vi "Termo_1.5__.vi"() -> ()   [LabVIEW 2013]
doc: "Программа мониторинга температуры"
uses:
  <vilib>/Utility/error.llb/DialogType.ctl
  Global R.vi
  Global T.vi
  Global P.vi
  PV ActiveLine/PV ActiveLine.lvlib
panel:
  out "Sensor 2":dbl format="%.3e"
  out "Sensor 1":dbl format="%.3e"
  in  "TPG COM port":refnum<visa-resource-name> caption="Eingang (Referenz)"
  in  "Интервал сохр. в файл, мин":u32=2 caption="Интервал сохр. в файл"
  out "Err":string=" INSTRUCTIONS:\r\rNormal Use:  When using subVIs that incorporate the error in/error out (or error I/O) structure, place this handler where you want to inform the user of an error, typically at the end of the I/O data path, as the last action of the program.  If the error in error? is ERROR, the handler creates a message describing the error and its source.  If the type of dialog = 1 (default), the message is displayed to the user, who can only acknowedge it.  If the type = 2, the user can acknowledge the message or abort execution; aborting a program with active I/O is not recommended.  If the type = 0, no message is displayed; this is used to process the error programmatically, and the error out cluster elements are wired to individual terminals for that reason.  \r\rOther Use:\n\r\nlocal testing.  To test the error code of a subVI or function that does not have the error I/O structure, you can wire its error code and a source string to the local error code and error source inputs.  If error in error? indicates no error and error code is not equal to 0, the local code and source are substituted for the error in values, and error? is set TRUE (ERROR)."
  out "Status Sensor 2":i32(ring) items=["data OK", "underrange", "overrange", "sensor error", "sensor off", "no sensor", "ID error"]
  out "Status Sensor 1":i32(ring) items=["data OK", "underrange", "overrange", "sensor error", "sensor off", "no sensor", "ID error"]
  in  "T13 koeff.":T1={"k1"=26.4009671199601144, "k2"=-324.931044271681458, "k3"=1711.37684206105769, "k4"=-4392.68239063024521, "k5"=6058.41654951870441, "k6"=-3986.95889506489038, "k7"=1183.01099493727087997} {"k7" format="%#_18g"; "k6" format="%#_18g"; "k5" format="%#_18g"; "k4" format="%#_18g"; "k3" format="%#_18g"; "k2" format="%#_18g"; "k1" format="%#_18g"}
  in  "T12 koeff.":T1={"k1"=17.07349405885907, "k2"=-214.441047532483935, "k3"=1210.98502247408031995, "k4"=-3244.2372938580811, "k5"=4710.0469546467065798, "k6"=-3214.85599070042372, "k7"=997.561462182551622} {"k7" format="%#_18g"; "k6" format="%#_18g"; "k5" format="%#_18g"; "k4" format="%#_18g"; "k3" format="%#_18g"; "k2" format="%#_18g"; "k1" format="%#_18g"}
  in  "T11 koeff.":T1={"k1"=23.375991559296380701, "k2"=-279.282885558437556, "k3"=1443.09818702377379, "k4"=-3601.37313615530729, "k5"=4833.89744386076927, "k6"=-3091.9414890073239801, "k7"=931.25663803331553903} {"k7" format="%#_18g"; "k6" format="%#_18g"; "k5" format="%#_18g"; "k4" format="%#_18g"; "k3" format="%#_18g"; "k2" format="%#_18g"; "k1" format="%#_18g"}
  in  "T10 koeff.":T1={"k1"=14.2047637495270465, "k2"=-178.266357081010938, "k3"=1036.21158173121512, "k4"=-2804.05543357878923, "k5"=4109.27601800113916, "k6"=-2758.27630065754056, "k7"=841.102514177560806} {"k7" format="%#_18g"; "k6" format="%#_18g"; "k5" format="%#_18g"; "k4" format="%#_18g"; "k3" format="%#_18g"; "k2" format="%#_18g"; "k1" format="%#_18g"}
  in  "T8 koeff.":T1={"k1"=22.4768360081361607, "k2"=-287.193510523065925, "k3"=1596.74034120887518, "k4"=-4282.5984272807836502, "k5"=6172.9084560498595202, "k6"=-4207.9212595894932698, "k7"=1298.64862929470837005} {"k7" format="%#_18g"; "k6" format="%#_18g"; "k5" format="%#_18g"; "k4" format="%#_18g"; "k3" format="%#_18g"; "k2" format="%#_18g"; "k1" format="%#_18g"}
  in  "T7 koeff.":T1={"k1"=22.696802702761488001, "k2"=-226.07392810517922, "k3"=970.613756582140923, "k4"=-1955.80814630538225, "k5"=2022.28153763338923, "k6"=-904.462546051479876, "k7"=215.64549227920360901} {"k7" format="%#_18g"; "k6" format="%#_18g"; "k5" format="%#_18g"; "k4" format="%#_18g"; "k3" format="%#_18g"; "k2" format="%#_18g"; "k1" format="%#_18g"}
  in  "T6 koeff.":T1={"k1"=28.2578839106718078, "k2"=-358.860014421865344, "k3"=1945.6722907833755, "k4"=-5171.24013045430183, "k5"=7400.41584329307079, "k6"=-5088.91018018126488, "k7"=1538.68586002103984} {"k7" format="%#_18g"; "k6" format="%#_18g"; "k5" format="%#_18g"; "k4" format="%#_18g"; "k3" format="%#_18g"; "k2" format="%#_18g"; "k1" format="%#_18g"}
  in  "T5 koeff.":T1={"k1"=11.9987486686586634996, "k2"=-140.311366179957986, "k3"=706.404515956528485, "k4"=-1587.81046432070434005, "k5"=1758.85326032713056, "k6"=-724.664392888546, "k7"=148.42783740232699} {"k7" format="%#_18g"; "k6" format="%#_18g"; "k5" format="%#_18g"; "k4" format="%#_18g"; "k3" format="%#_18g"; "k2" format="%#_18g"; "k1" format="%#_18g"}
  in  "T4 koeff.":T1={"k1"=35.418606627499684698, "k2"=-55510.2443863153458, "k3"=36541155.640991210901, "k4"=-11725993248.921875, "k5"=1971553990780.0, "k6"=-153283011720960.0, "k7"=5052534013419520.0} {"k7" format="%#_18g"; "k6" format="%#_18g"; "k5" format="%#_18g"; "k4" format="%#_18g"; "k3" format="%#_18g"; "k2" format="%#_18g"; "k1" format="%#_18g"}
  in  "T3 koeff.":T1={"k1"=25.230552436260040799, "k2"=-268.022426915355027, "k3"=1234.06186301074921996, "k4"=-2752.2769357189536099, "k5"=3276.3375887721777, "k6"=-1820.06986418552697, "k7"=447.66889524366706599} {"k7" format="%#_18g"; "k6" format="%#_18g"; "k5" format="%#_18g"; "k4" format="%#_18g"; "k3" format="%#_18g"; "k2" format="%#_18g"; "k1" format="%#_18g"}
  in  "T2 koeff.":T1={"k1"=21.575617982307449, "k2"=-260.23302811570465001, "k3"=1369.9472036678344, "k4"=-3472.20134520530701, "k5"=4749.71195641905069, "k6"=-3111.58472899347544, "k7"=957.900049353018403} {"k7" format="%#_18g"; "k6" format="%#_18g"; "k5" format="%#_18g"; "k4" format="%#_18g"; "k3" format="%#_18g"; "k2" format="%#_18g"; "k1" format="%#_18g"}
  in  "T1 koeff.":T1={"k1"=16.924520218221005099, "k2"=-209.88193494221195599, "k3"=1166.48439995385706, "k4"=-3075.28152279928327, "k5"=4388.5694366171956098, "k6"=-2910.95083422213793, "k7"=868.100233905948699} {"k7" format="%#_18g"; "k6" format="%#_18g"; "k5" format="%#_18g"; "k4" format="%#_18g"; "k3" format="%#_18g"; "k2" format="%#_18g"; "k1" format="%#_18g"}
  out "R16":dbl format="%.2f"
  out "R15":dbl format="%.2f"
  out "PKT2 updated":bool=TRUE
  out "PKT1 updated":bool=TRUE
  out "ПКТ2-R":T2
  out "ПКТ2-T":T2
  out "ПКТ1-T":T2
  out "ПКТ1-R":T2
  in  "Графики N температур":bool
  in  "4 K gr":bool
  in  "Tab Control":enum32{"Измерения", "Настройки"}(tab)
  in  "stop":bool
  out "R9":dbl format="%.2f"
  out "R10":dbl format="%.2f"
  out "R11":dbl format="%.2f"
  out "R12":dbl format="%.2f"
  out "R13":dbl format="%.2f"
  out "R14":dbl format="%.2f"
  out "R7":dbl format="%.2f"
  out "R5":dbl format="%.2f"
  out "R8":dbl format="%.2f"
  out "R6":dbl format="%.2f"
  out "R3":dbl format="%.2f"
  out "R1":dbl format="%.2f"
  out "R4":dbl format="%.2f"
  out "R2":dbl format="%.2f"
  in  "GraphLookB":bool
  in  "Старт измер.":bool
  in  "Стоп измер.":bool
  in  "IP-адрес 2":string="192.168.127.102"
  in  "порт 2":u16=4001
  in  "connect 2":bool
  in  "disconnect 2":bool
  in  "порт":u16=4001
  in  "IP-адрес":string="192.168.127.101"
  in  "connect":bool
  in  "disconnect":bool
  in  "SPS":T3(ring)
  in  "Buf_size":u8=16 min=1 max=128
  in  "ADC_dyn_range":T4(ring)=enum."± 0.625 В"
  out "Связь с прибором":bool
  out "Связь с прибором 2":bool
  out "Т7":dbl format="%.2f"
  out "Т1":dbl format="%.2f"
  out "T12":dbl format="%.2f"
  out "T10":dbl format="%.2f"
  out "T9":dbl format="%.2f"
  out "T11":dbl format="%.2f"
  out "T13":dbl format="%.2f"
  out "T14":dbl format="%.2f"
  out "Т8":dbl format="%.2f"
  out "Т6":dbl format="%.2f"
  out "Т5":dbl format="%.2f"
  out "T4":dbl format="%.2f"
  out "Т2":dbl format="%.2f"
  out "Т3":dbl format="%.2f"
  out "T15":dbl format="%.2f"
  out "T16":dbl format="%.2f"
  out "connection ID 2":refnum<k5>
  out "disconnected 2":bool
  out "Расположение\n файла":path caption="Расположение файла"
  in  "load_coeff.":bool caption="Disconn"
  in  "save_coeff.":bool caption="Disconn"
  out "Configuring ADC?":bool
  in  "Запись в файл":bool
  out "refnum out":refnum<file>
  in  "File header exist?":bool caption="Disconn"
  out "connection ID":refnum<k5>
  out "Расположение файла":path
  # "КРИОН-Т"
  # "4 K"
  # "40 K"
  # "P"
  # "mBar"
  # "мин."
  # "Измерения"
  # "R [Ом]"
  # "R1"
  # "R2"
  # "R3"
  # "R4"
  # "R5"
  # "R6"
  # "R7"
  # "R8"
  # "R9"
  # "R10"
  # "R11"
  # "R12"
  # "R13"
  # "R14"
  # "Скорость измерений"
  # "SPS = Samples Per Second"
  # "Динамический диапазон"
  # "Размер буфера усреднения"
  # "Подключение"
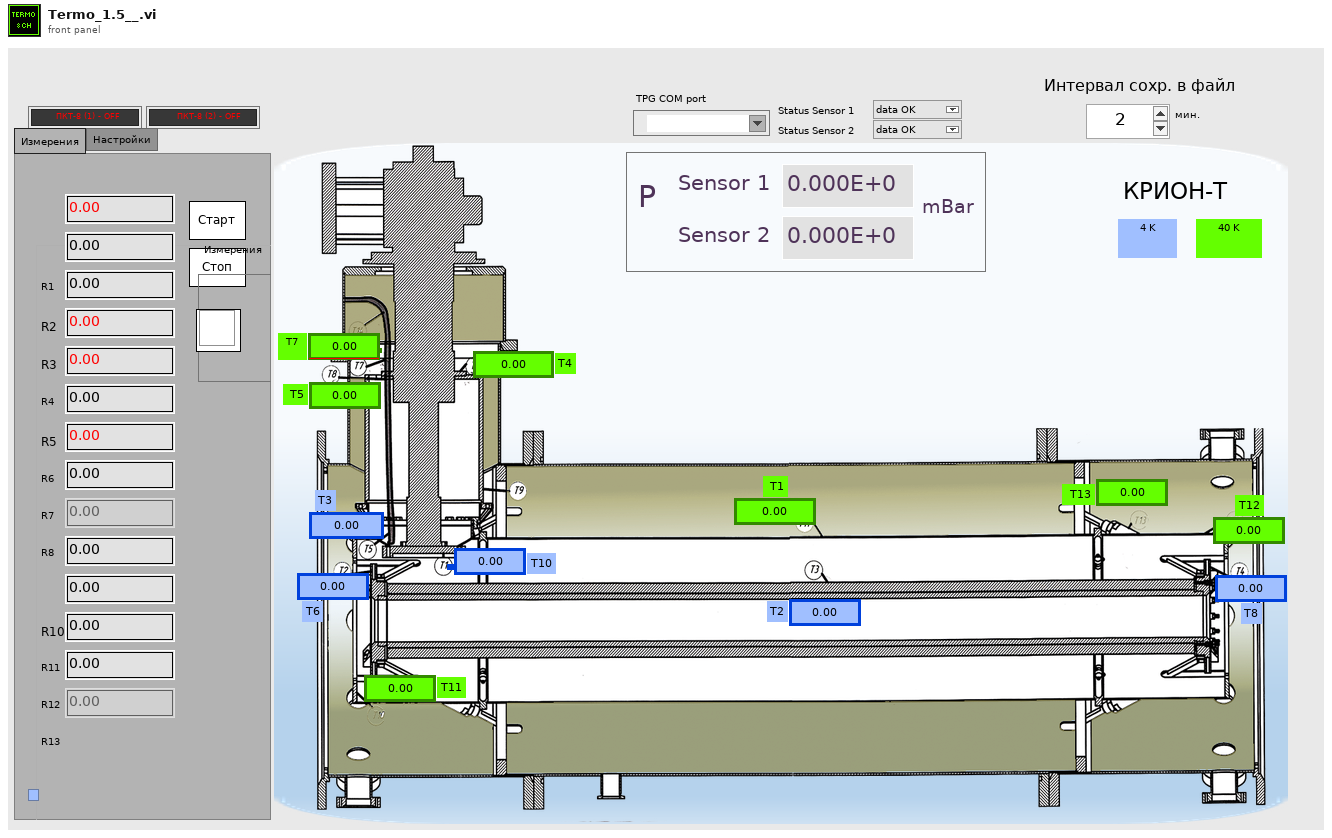
[diagram p1: front panel]
types:
  T1 = cluster{"k1":ext, "k2":ext, "k3":ext, "k4":ext, "k5":ext, "k6":ext, "k7":ext}
  T2 = cluster{" R1":dbl, " R2":dbl, " R3":dbl, " R4":dbl, " R5":dbl, "R6":dbl, " R7":dbl, "R8":dbl}
  T3 = enum16{"2,5 SPS", "5 SPS", "10 SPS", "25 SPS", "50 SPS", "100 SPS", "500 SPS", "1 kSPS", "3,75 kSPS"}
  T4 = enum16{"± 5 В", "± 2.5 В", "± 1.25 В", "± 0.625 В", "± 312.5 мВ", "± 156.25 мВ", "± 78.125 мВ"}
  T5 = enum32{"Page Enabled", "Page Disabled", "Page Disabled & Grayed"}
  T6 = typedef "DialogType.ctl" = u16
  T7 = enum16{"Standard", "Buffered", "CRLF", "Immediate"}
  T8 = cluster{"Pressure Sensor 1":dbl, "Pressure Sensor 2":dbl}
  T9 = cluster{" R9":dbl, " R10":dbl, " R11":dbl, " R12":dbl, " R13":dbl, "R14":dbl, "R15":dbl, "R16":dbl}
  T10 = cluster{" T9":dbl, "T10":dbl, "T11":dbl, "T12":dbl, " T13":dbl, "T14":dbl, "T15":dbl, "T16":dbl}
  T11 = cluster{" R1":dbl, " R2":dbl, " R3":dbl, " R4":dbl, " R5":dbl, "R6":dbl, " R7":dbl, "R8":dbl, " R1":dbl, " R2":dbl, " R3":dbl, " R4":dbl, " R5":dbl, "R6":dbl, " R7":dbl, "R8":dbl}
  T12 = cluster{" Т1":dbl, "Т2":dbl, "Т3":dbl, "T4":dbl, " Т5":dbl, "Т6":dbl, "Т7":dbl, "Т8":dbl}
  T13 = enum32{"Invalid", "Standard", "Closed", "Hidden", "Minimized", "Maximized"}
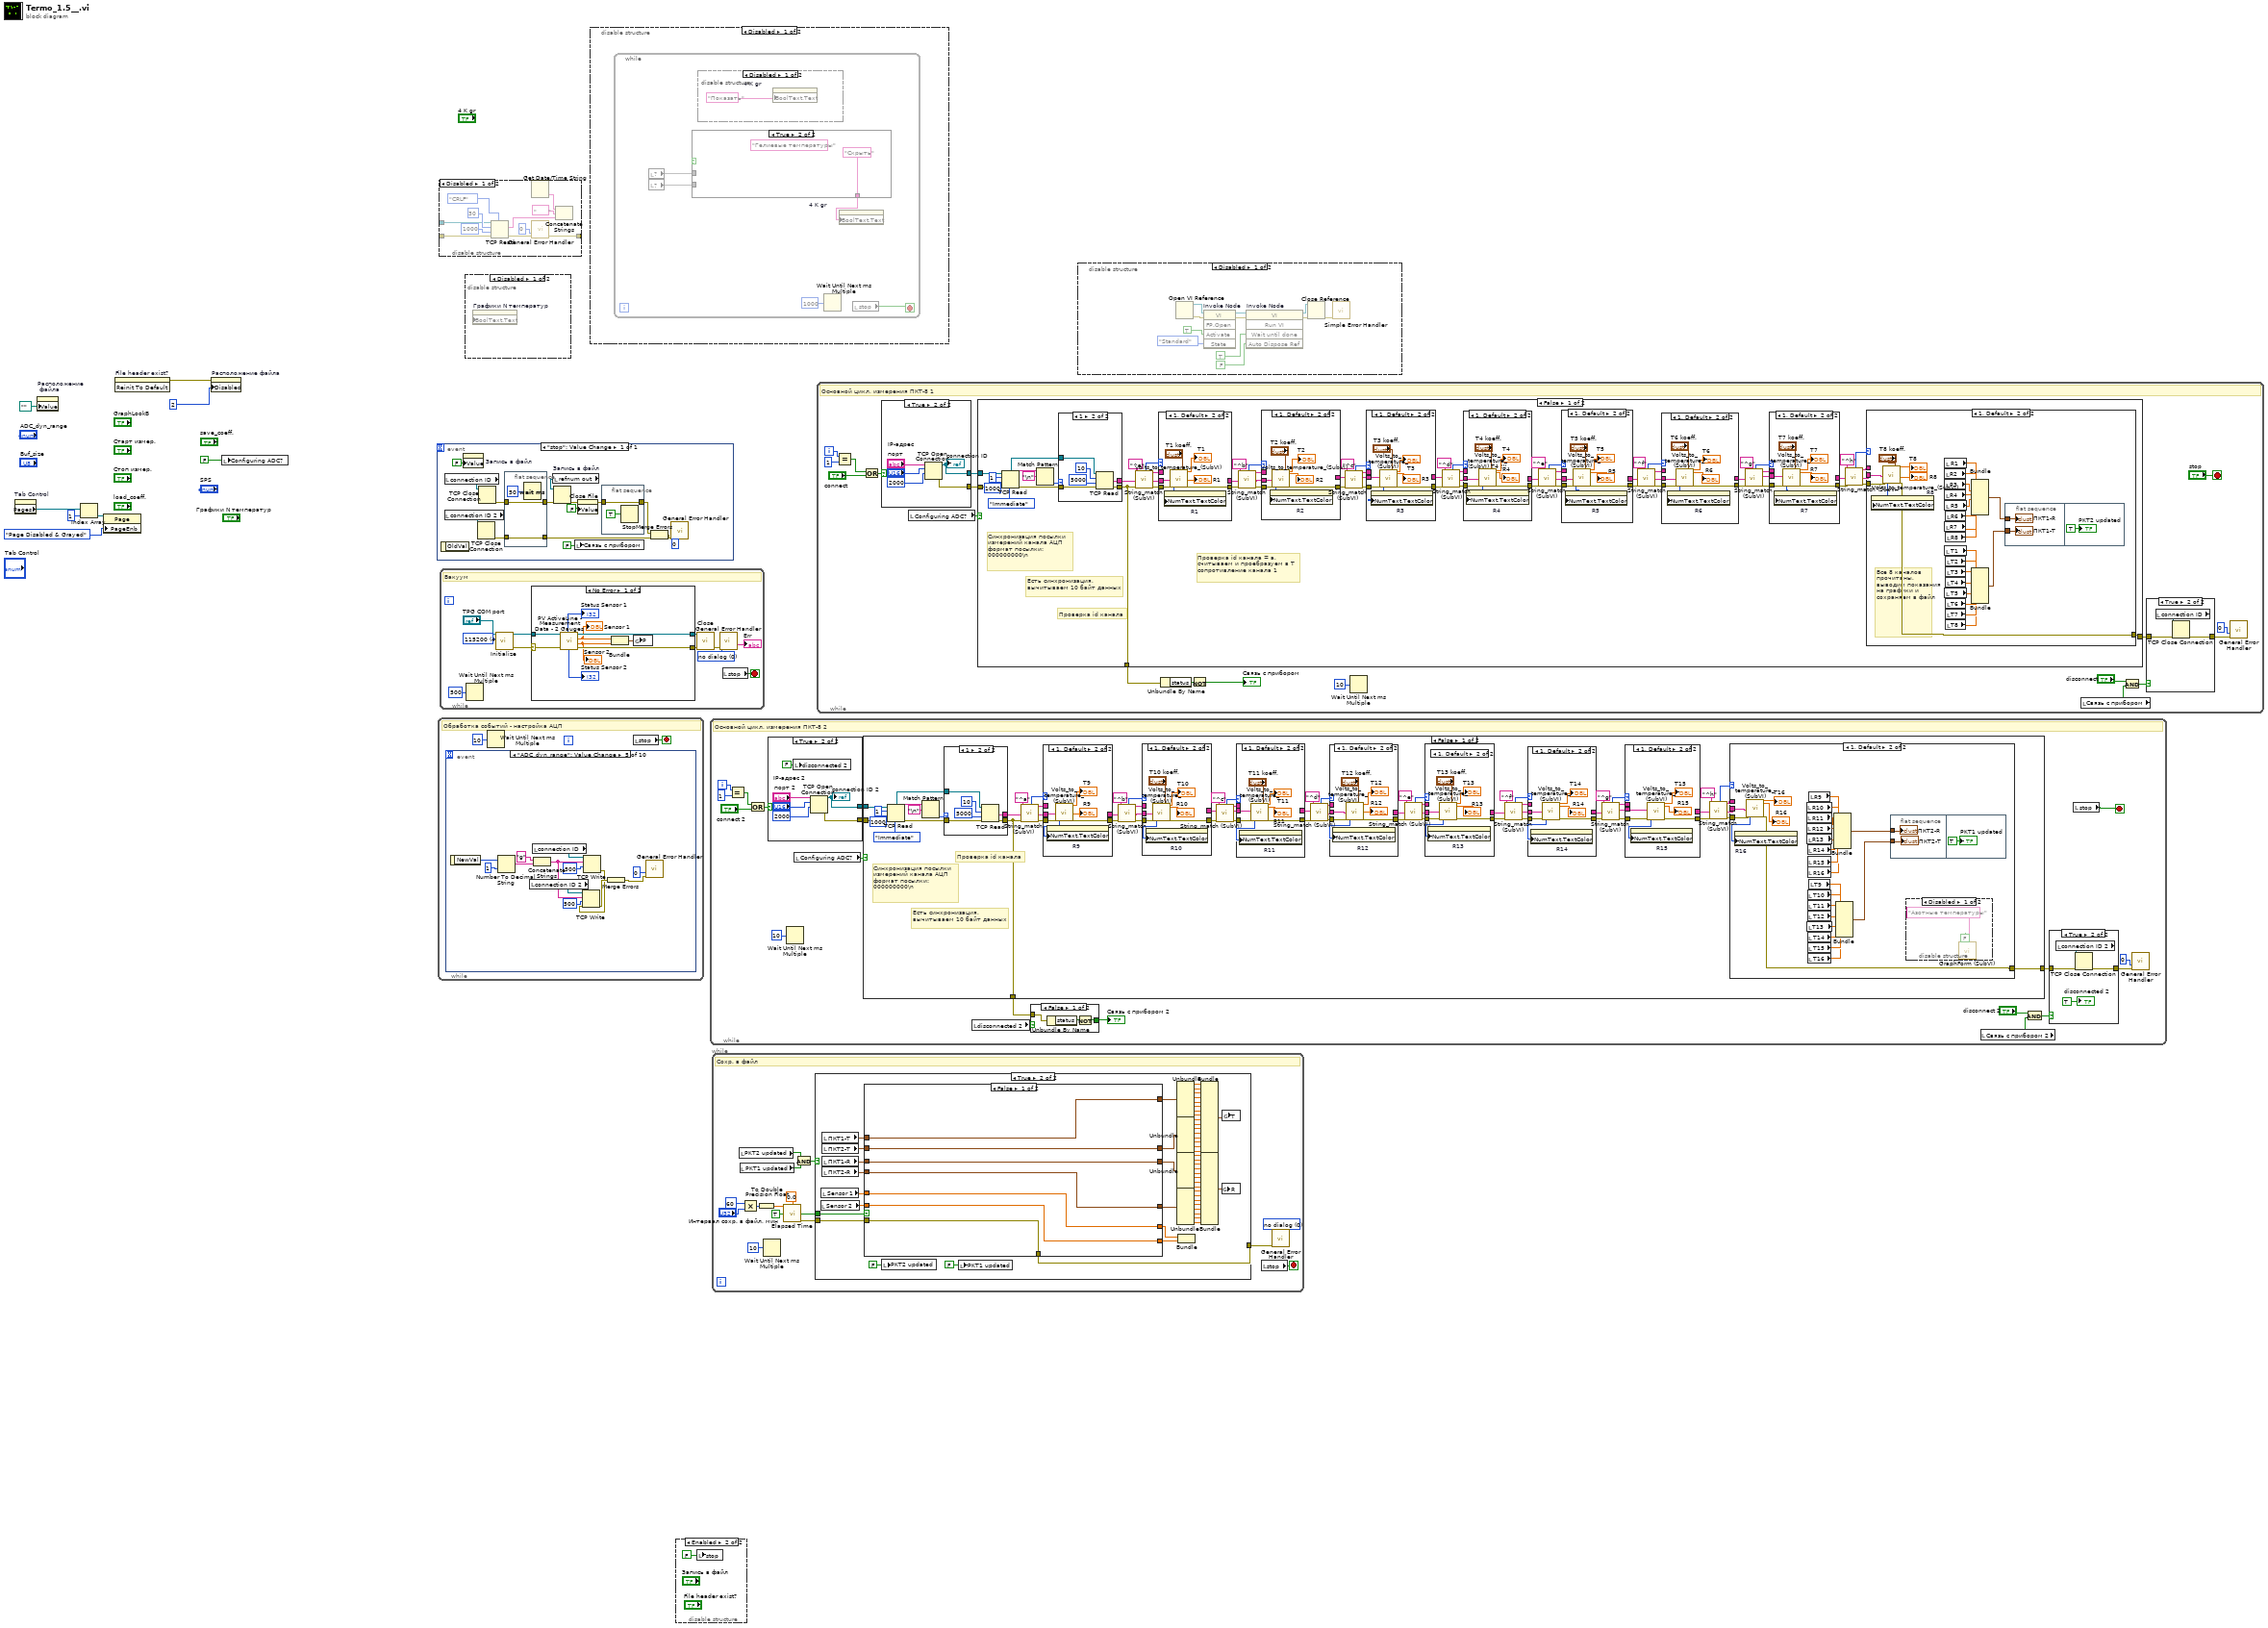
[diagram p0: block diagram]
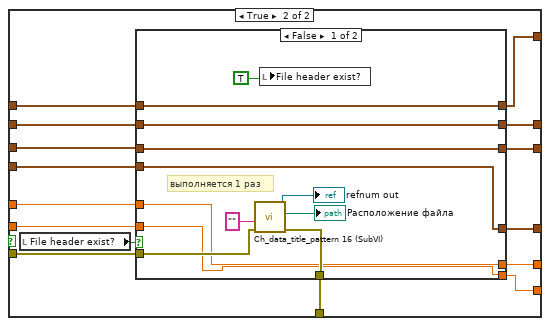
[diagram p3: hidden frame]
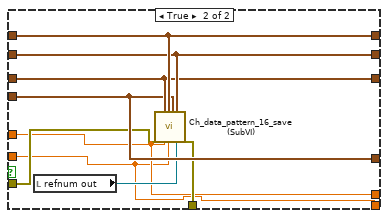
[diagram p4: hidden frame]
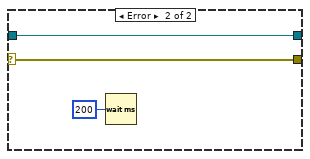
[diagram p5: hidden frame]
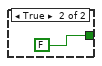
[diagram p8: hidden frame]
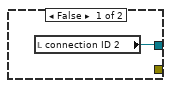
[diagram p10: hidden frame]
diagram:
  n1 = property on="Tab Control" class="TabCtl (strict)"() -> ("Pages"=w1:refnum<vi>[])  [unwired: 2 in, 2 out]
  n2 = property on="Расположение\n файла" class="Path"("Value"=path "" ("Расположение\n файла")) -> ()  [unwired: 2 in, 2 out]
  n3 = Index Array(array=w1, index=1) -> (element=w3:refnum<vi>)
  n4 = property class="Page"(reference=w3, "PageEnb"=T5."Page Disabled & Grayed" ("Page Enabled State")) -> ()  [unwired: 1 in, 2 out]
  n5 = invoke on="File header exist?" class="Bool (strict)" method="Reinit To Default"() -> (error out=w7:errorcluster)  [unwired: 3 in, 2 out]
  n6 = property on="Расположение файла" class="Path"(error in=w7, "Disabled"=u8 2) -> ()  [unwired: 1 in, 2 out]
  n7 = local write "Configuring ADC?"(FALSE ("TCP_Wr_fl")) -> ()
  n8 = event shown="[0] \"stop\": Value Change" {
    selector: _ -> [_]
    dyn-events: _ -> [_]
    timeout: _ -> [_]
    event "stop": Value Change {
      (unwired) 0 ("timeout ms (25000)")
      n9 = event-data() -> ()  [unwired: 1 in, 1 out]
      n10 = local read "connection ID"() -> (w17:refnum<k5>)
      n11 = local read "connection ID 2"() -> (w15:refnum<k5>)
      n12 = property on="Запись в файл" class="Bool (strict)"("Value"=FALSE ("Запись в файл")) -> ()  [unwired: 2 in, 2 out]
      n13 = TCP Close Connection(connection ID=w15) -> (error out=w14:errorcluster)  [unwired: 1 in, 2 out]
      n14 = TCP Close Connection(connection ID=w17) -> (error out=w22:errorcluster)  [unwired: 1 in, 2 out]
      n15 = flat-sequence {
        tunnel: [w26] -> w12
        tunnel: w22 -> [w26]
        tunnel: [w25] -> w11
        tunnel: w14 -> [w25]
        frame #0 {
          n16 = Wait (ms)(milliseconds to wait=u32 50) -> ()  [unwired: 1 out]
        }
      }
      n17 = local read "refnum out"() -> (w19:refnum<file>)
      n18 = Close File(refnum=w19, error in=w12) -> (error out=w18:errorcluster)  [unwired: 1 out]
      n19 = local write "Связь с прибором"(FALSE ("Запись в файл")) -> ()
      n20 = property on="Запись в файл" class="Bool (strict)"(error in=w18, "Value"=FALSE ("Запись в файл")) -> (error out=w16:errorcluster)  [unwired: 1 in, 1 out]
      n21 = flat-sequence {
        tunnel: w16 -> [w24]
        tunnel: [w24] -> w10
        frame #0 {
          n22 = Stop(stop? (T)=TRUE) -> ()
        }
      }
      n23 = Merge Errors(w10, w11) -> (w13:errorcluster)
      n24 = call <vilib>:"General Error Handler.vi"("error in (no error)"=w13) -> ()  [unwired: 10 in, 5 out]
    }
  }
  n25 = while {
    stop <- w28 stop-if-true
    # "Обработка событий - настройка АЦП"
    n26 = event shown="[4] \"ADC_dyn_range\": Value Change" {
      selector: _ -> [_ _ _ _ _ _ _ _ _ _]
      dyn-events: _ -> [_ _ _ _ _ _ _ _ _ _]
      timeout: _ -> [_ _ _ _ _ _ _ _ _ _]
      event "Старт измер.": Value Change {
        w37 = 0.0 ("3")
        w41 = 0.0 ("3")
        n27 = event-data() -> ("OldVal"=w49:bool)  [unwired: 1 in]
        n28 = local write "Старт измер."(w49) -> ()
        n29 = local read "connection ID"() -> (w45:refnum<k5>)
        n30 = local read "connection ID 2"() -> (w36:refnum<k5>)
        n31 = property on="Tab Control" class="TabCtl (strict)"() -> (error out=w39:errorcluster, "Pages"=w38:refnum<vi>[])  [unwired: 2 in, 1 out]
        n32 = Index Array(array=w38, index=1) -> (element=w44:refnum<vi>)
        n33 = local write "R3"(w41) -> ()
        n34 = local write "R8"(w41) -> ()
        n35 = local write "R1"(w41) -> ()
        n36 = local write "R6"(w41) -> ()
        n37 = local write "R4"(w41) -> ()
        n38 = local write "R2"(w41) -> ()
        n39 = local write "R5"(w41) -> ()
        n40 = local write "R7"(w41) -> ()
        n41 = property class="Page"(reference=w44, error in=w39, "PageEnb"=T5."Page Disabled & Grayed" ("Page Enabled State")) -> (error out=w32:errorcluster)  [unwired: 1 out]
        n42 = TCP Write(connection ID=w45, data in="s", 9:500 ("timeout ms (25000)")) -> (error out=w30:errorcluster)  [unwired: 1 in, 2 out]
        n43 = TCP Write(connection ID=w36, data in="s", error in (no error)=w30, 9:500 ("timeout ms (25000)")) -> (error out=w33:errorcluster)  [unwired: 2 out]
        n44 = local write "R10"(w37) -> ()
        n45 = local write "R11"(w37) -> ()
        n46 = local write "R12"(w37) -> ()
        n47 = local write "R13"(w37) -> ()
        n48 = local write "R14"(w37) -> ()
        n49 = local write "R15"(w37) -> ()
        n50 = local write "R16"(w37) -> ()
        n51 = local write "R9"(w37) -> ()
        n52 = Merge Errors(w33, w32) -> (w31:errorcluster)
        n53 = call <vilib>:"General Error Handler.vi"("type of dialog (OK msg:1)"=0 ("timeout ms (25000)"), "error in (no error)"=w31) -> ()  [unwired: 9 in, 5 out]
        "Configuring ADC?" <- FALSE ("TCP_Wr_fl")
      }
      event "Стоп измер.": Value Change {
        n54 = event-data() -> ("OldVal"=w67:bool)  [unwired: 1 in]
        n55 = local read "connection ID 2"() -> (w58:refnum<k5>)
        n56 = property on="Tab Control" class="TabCtl (strict)"() -> (error out=w51:errorcluster, "Pages"=w59:refnum<vi>[])  [unwired: 2 in, 1 out]
        n57 = local read "connection ID"() -> (w64:refnum<k5>)
        n58 = local write "Configuring ADC?"(TRUE ("TCP_Wr_fl")) -> ()
        n59 = local write "Стоп измер."(w67) -> ()
        n60 = Index Array(array=w59, index=1) -> (element=w62:refnum<vi>)
        n61 = property class="Page"(reference=w62, error in=w51, "PageEnb"=T5."Page Enabled" ("Page Enabled State")) -> (error out=w52:errorcluster)  [unwired: 1 out]
        n62 = TCP Write(connection ID=w64, data in="p", 9:500 ("timeout ms (25000)")) -> (error out=w50:errorcluster)  [unwired: 1 in, 2 out]
        n63 = TCP Write(connection ID=w58, data in="p", error in (no error)=w50, 9:500 ("timeout ms (25000)")) -> (error out=w53:errorcluster)  [unwired: 2 out]
        n64 = Merge Errors(w53, w52) -> (w54:errorcluster)
        n65 = call <vilib>:"General Error Handler.vi"("type of dialog (OK msg:1)"=0 ("timeout ms (25000)"), "error in (no error)"=w54) -> ()  [unwired: 9 in, 5 out]
      }
      event "SPS": Value Change {
        n66 = event-data() -> ("NewVal"=w76:T3)  [unwired: 1 in]
        n67 = Number To Decimal String(number=w76, width (-)=i16 1) -> (decimal integer string=w74:string)
        n68 = Concatenate Strings("v" ("data in"), w74) -> (w70:string)
        n69 = local read "connection ID 2"() -> (w72:refnum<k5>)
        n70 = local read "connection ID"() -> (w78:refnum<k5>)
        n71 = TCP Write(connection ID=w78, data in=w70, 9:500 ("timeout ms (25000)")) -> (error out=w69:errorcluster)  [unwired: 1 in, 2 out]
        n72 = TCP Write(connection ID=w72, data in=w70, error in (no error)=w69, 9:500 ("timeout ms (25000)")) -> (error out=w68:errorcluster)  [unwired: 2 out]
        n73 = call <vilib>:"General Error Handler.vi"("type of dialog (OK msg:1)"=0 ("timeout ms (25000)"), "error in (no error)"=w68) -> ()  [unwired: 9 in, 5 out]
      }
      event "Buf_size": Value Change {
        n74 = event-data() -> ("NewVal"=w94:u8)  [unwired: 1 in]
        n75 = Number To Decimal String(number=w94, width (-)=i16 3) -> (decimal integer string=w92:string)
        n76 = Concatenate Strings("b" ("data in"), w92) -> (w91:string)
        n77 = call <vilib>:"Space Constant.vi"() -> ("String"=w90:string)
        n78 = Search and Replace String(replace all?=TRUE ("replace all? (F)"), input string=w91, search string=w90, replace string="0" ("replace string (\"\")")) -> (result string=w81:string, error out=w87:errorcluster)  [unwired: 4 in, 2 out]
        n79 = local read "connection ID 2"() -> (w85:refnum<k5>)
        n80 = local read "connection ID"() -> (w96:refnum<k5>)
        n81 = TCP Write(connection ID=w96, data in=w81, error in (no error)=w87, 9:500 ("timeout ms (25000)")) -> (error out=w80:errorcluster)  [unwired: 2 out]
        n82 = TCP Write(connection ID=w85, data in=w81, error in (no error)=w80, 9:500 ("timeout ms (25000)")) -> (error out=w83:errorcluster)  [unwired: 2 out]
        n83 = Merge Errors(w83) -> (w82:errorcluster)
        n84 = call <vilib>:"General Error Handler.vi"("type of dialog (OK msg:1)"=0 ("timeout ms (25000)"), "error in (no error)"=w82) -> ()  [unwired: 9 in, 5 out]
      }
      event "ADC_dyn_range": Value Change {
        n85 = event-data() -> ("NewVal"=w107:T4)  [unwired: 1 in]
        n86 = Number To Decimal String(number=w107, width (-)=i16 1) -> (decimal integer string=w105:string)
        n87 = local read "connection ID 2"() -> (w103:refnum<k5>)
        n88 = local read "connection ID"() -> (w109:refnum<k5>)
        n89 = Concatenate Strings("g" ("data in"), w105) -> (w99:string)
        n90 = TCP Write(connection ID=w109, data in=w99, 9:500 ("timeout ms (25000)")) -> (error out=w98:errorcluster)  [unwired: 1 in, 2 out]
        n91 = TCP Write(connection ID=w103, data in=w99, error in (no error)=w98, 9:500 ("timeout ms (25000)")) -> (error out=w101:errorcluster)  [unwired: 2 out]
        n92 = Merge Errors(w101) -> (w100:errorcluster)
        n93 = call <vilib>:"General Error Handler.vi"("type of dialog (OK msg:1)"=0 ("timeout ms (25000)"), "error in (no error)"=w100) -> ()  [unwired: 9 in, 5 out]
      }
      event "save_coeff.": Value Change {
        w111 = T6 0 items=["no dialog", "OK message", "continue or stop message", "OK message + warnings", "continue/stop + warnings"] ("type of dialog (OK msg:1)")
        n94 = event-data() -> ("OldVal"=w115:bool)  [unwired: 1 in]
        n95 = call "Cluster_to_string_(SubVI).vi"() -> ("string of coefficients"=w119:string, "error out"=w114:errorcluster)  [unwired: 14 in]
        n96 = call "Cluster_to_string_(SubVI).vi"() -> ("string of coefficients"=w120:string, "error out"=w113:errorcluster)  [unwired: 14 in]
        n97 = local write "save_coeff."(w115) -> ()
        n98 = Concatenate Strings(w119, w120) -> (w116:string)
        n99 = Merge Errors(w114, w113) -> (w118:errorcluster)
        n100 = call "Create_and_save_to_file (SubVI).vi"("input string"=w116, "error in"=w118) -> ("Текущее расположение файла"=→"Расположение\n файла":path, "error out"=w112:errorcluster)  [unwired: 4 in]
        n101 = call <vilib>:"General Error Handler.vi"("type of dialog (OK msg:1)"=w111, "error in (no error)"=w112) -> ()  [unwired: 9 in, 5 out]
      }
      event "load_coeff.": Value Change {
        w122 = T6 0 items=["no dialog", "OK message", "continue or stop message", "OK message + warnings", "continue/stop + warnings"] ("type of dialog (OK msg:1)")
        n102 = event-data() -> ("OldVal"=w128:bool)  [unwired: 1 in]
        n103 = Read from Text File(prompt (Open existing file)="Укажите  файл с коэффициентами...") -> (refnum out=w121:refnum<file>, text=w125:string, cancelled=w124:bool, error out=w126:errorcluster)  [unwired: 3 in]
        n104 = case shown="False" w124 {
          tunnel: w126 -> [w140 w141]
          tunnel: w125 -> [w139 _]
          tunnel: [w129 w141] -> w123
          tunnel: w121 -> [w131 _]
          frame False {
            n105 = call "String_to_num (SubVI).vi"("String in"=w139, "error in"=w140) -> ("Rest of string OUT"=w138:string)  [unwired: 5 in, 2 out]
            n106 = Refnum to Path(1:w131) -> (0:w130:path)
            n107 = call "String_to_num (SubVI).vi"("String in"=w138) -> ("Rest of string OUT"=w137:string)  [unwired: 6 in, 2 out]
            n108 = call "String_to_num (SubVI).vi"("String in"=w137) -> ("Rest of string OUT"=w136:string)  [unwired: 6 in, 2 out]
            n109 = local write "Расположение\n файла"(w130) -> ()
            n110 = call "String_to_num (SubVI).vi"("String in"=w136) -> ("Rest of string OUT"=w135:string)  [unwired: 6 in, 2 out]
            n111 = call "String_to_num (SubVI).vi"("String in"=w135) -> ("Rest of string OUT"=w134:string)  [unwired: 6 in, 2 out]
            n112 = call "String_to_num (SubVI).vi"("String in"=w134) -> ("Rest of string OUT"=w133:string)  [unwired: 6 in, 2 out]
            n113 = call "String_to_num (SubVI).vi"("String in"=w133) -> ("Rest of string OUT"=w132:string)  [unwired: 6 in, 2 out]
            n114 = call "String_to_num (SubVI).vi"("String in"=w132) -> ("error out"=w129:errorcluster)  [unwired: 6 in, 2 out]
          }
          frame True {
          }
        }
        n115 = local write "load_coeff."(w128) -> ()
        n116 = call <vilib>:"General Error Handler.vi"("type of dialog (OK msg:1)"=w122, "error in (no error)"=w123) -> ()  [unwired: 9 in, 5 out]
      }
      event "GraphLookB": Value Change {
        n117 = event-data() -> ()  [unwired: 1 in, 1 out]
        n118 = control-ref of="This VI"() -> (w142:refnum<vi>)
        n119 = local write "GraphLookB"(FALSE ("Снимок")) -> ()
        n120 = call "CheckScreenShot (SubVI).vi"("VI reference"=w142) -> ()  [unwired: 15 in]
      }
      event "4 K gr": Value Change {
        n121 = event-data() -> ()  [unwired: 1 in, 1 out]
      }
      event Panel Close? {
        n122 = event-data() -> ()  [unwired: 1 in, 1 out]
        n123 = Two Button Dialog(message="Действительно закрыть?", 1:"Отмена" ("T button name (\"OK\")"), 2:"Да" ("T button name (\"OK\")")) -> (T button?=w148:bool)
        n124 = case shown="True" w148 {
          tunnel: [TRUE ("Discard?") FALSE ("Discard?")] -> w144
          frame False {
          }
          frame True {
            (unwired) 0 ("timeout ms (25000)")
            n125 = local read "connection ID 2"() -> (w156:refnum<k5>)
            n126 = local read "connection ID"() -> (w158:refnum<k5>)
            n127 = local read "refnum out"() -> (w160:refnum<file>)
            n128 = property on="Запись в файл" class="Bool (strict)"("Value"=FALSE ("Запись в файл")) -> ()  [unwired: 2 in, 2 out]
            n129 = local write "Связь с прибором"(FALSE ("Запись в файл")) -> ()
            n130 = Close File(refnum=w160) -> (error out=w159:errorcluster)  [unwired: 1 in, 1 out]
            n131 = property on="Запись в файл" class="Bool (strict)"(error in=w159, "Value"=FALSE ("Запись в файл")) -> (error out=w151:errorcluster)  [unwired: 1 in, 1 out]
            n132 = TCP Close Connection(connection ID=w158) -> (error out=w163:errorcluster)  [unwired: 1 in, 2 out]
            n133 = TCP Close Connection(connection ID=w156) -> (error out=w154:errorcluster)  [unwired: 1 in, 2 out]
            n134 = flat-sequence {
              tunnel: [w165] -> w155
              tunnel: w163 -> [w165]
              tunnel: w154 -> [w164]
              tunnel: [w164] -> w153
              frame #0 {
                n135 = Wait (ms)(milliseconds to wait=u32 50) -> ()  [unwired: 1 out]
              }
            }
            n136 = Merge Errors(w155, w153, w151) -> (w150:errorcluster)
            n137 = call <vilib>:"General Error Handler.vi"("error in (no error)"=w150) -> ()  [unwired: 10 in, 5 out]
          }
        }
        n138 = event-data("Discard?"=w144) -> ()  [unwired: 1 in, 1 out]
      }
    }
    n139 = Wait Until Next ms Multiple(millisecond multiple=u32 10) -> ()  [unwired: 1 out]
    n140 = local read "stop"() -> (w28:bool)
  }
  n141 = disable-structure shown="Disabled" {
    disable-tunnel: _ -> [w174 _]
    disable-tunnel: _ -> [w173 _]
    disable-tunnel: [w168 _] -> _
    frame Disabled {
      n142 = TCP Read(connection ID=w174, bytes to read=30, error in (no error)=w173, 7:T7."CRLF" ("mode (standard)"), 9:1000 ("timeout ms (25000)")) -> (data out=w170:string, error out=w169:errorcluster)  [unwired: 1 out]
      n143 = Get Date/Time String() -> (time string=w172:string)  [unwired: 3 in, 1 out]
      n144 = call <vilib>:"General Error Handler.vi"("type of dialog (OK msg:1)"=0 ("timeout ms (25000)"), "error in (no error)"=w169) -> ("error out"=w168:errorcluster)  [unwired: 9 in, 4 out]
      n145 = Concatenate Strings(w172, "      " ("string"), w170) -> ()  [unwired: 1 out]
    }
    frame Enabled {
    }
  }
  n146 = while {
    stop <- w185 stop-if-true
    w179 = u32 4 items=["9600 (default)", "19200", "38400", "57600", "115200"] ("Baud Rate")
    w183 = T6 0 items=["no dialog", "OK message", "continue or stop message", "OK message + warnings", "continue/stop + warnings"] ("type of dialog (OK msg:1)")
    # "Вакуум"
    n147 = Wait Until Next ms Multiple(millisecond multiple=u32 500) -> ()  [unwired: 1 out]
    n148 = call "Initialize.vi"("Baud Rate"=w179, "input refnum"="TPG COM port") -> ("Cluster (Ausgang)"=w181:errorcluster, "Referenz out"=w180:refnum<visa-resource-name>)  [unwired: 8 in]
    n149 = case shown="No Error" w181 {
      selector: w181 -> [w195 w200]
      tunnel: [w197 w198] -> w188
      tunnel: [w196 w200] -> w187
      tunnel: w180 -> [w192 w198]
      frame No Error {
        n150 = call "PV ActiveLine - Measurement Data - 2 Gauges.vi"("Fehler (Eingang)"=w195, "Referenz in"=w192) -> ("Cluster (Ausgang)"=w196:errorcluster, "Pressure Sensor 2"=w190:dbl, "Pressure Sensor 1"=w191:dbl, "Referenz out"=w197:refnum<visa-resource-name>, "Status Sensor 2"=→"Status Sensor 2":i32, "Status Sensor 1"=→"Status Sensor 1":i32)  [unwired: 4 in]
        "Sensor 1" <- w191
        "Sensor 2" <- w190
        n151 = Bundle("Pressure Sensor 1"=w191, "Pressure Sensor 2"=w190) -> (w189:T8)  [unwired: 1 in]
        n152 = global write "Global P.vi" "P"(w189) -> ()
      }
      frame Error {
        n153 = Wait (ms)(milliseconds to wait=u32 200) -> ()  [unwired: 1 out]
      }
    }
    n154 = call "Close.vi"("error in (no error)"=w187, "VISA resource name"=w188) -> ("error out"=w184:errorcluster)  [unwired: 9 in]
    n155 = call <vilib>:"General Error Handler.vi"("type of dialog (OK msg:1)"=w183, "error in (no error)"=w184) -> ("message"=→"Err":string)  [unwired: 9 in, 4 out]
    n156 = local read "stop"() -> (w185:bool)
  }
  n157 = disable-structure shown="Disabled" {
    frame Disabled {
      n158 = property on="Графики N температур" class="Bool (strict)" props=["BoolText", "Text"]() -> ()  [unwired: 3 in, 2 out]
    }
    frame Enabled {
    }
  }
  n159 = disable-structure shown="Disabled" {
    frame Disabled {
      n160 = while {
        i -> [w205]
        stop <- w207 stop-if-true
        n161 = local read item#-1() -> (w203)
        n162 = local read item#-1() -> (w202)
        n163 = case shown="True" w204 {
          tunnel: w203 -> [_ w211]
          tunnel: w202 -> [_ w210]
          tunnel: ["Показать" ("Boolean Text.Text") "Скрыть" ("Boolean Text.Text")] -> w201
          frame False {
          }
          frame True {
            w212 = "Гелиевые температуры" ("Title")
          }
        }
        n164 = disable-structure shown="Disabled" {
          frame Disabled {
            n165 = property on="4 K gr" class="Bool (strict)"("BoolText.Text"="Показать" ("Boolean Text.Text")) -> ()  [unwired: 2 in, 2 out]
          }
          frame Enabled {
          }
        }
        n166 = Wait Until Next ms Multiple(millisecond multiple=u32 1000) -> ()  [unwired: 1 out]
        n167 = property on="4 K gr" class="Bool (strict)"("BoolText.Text"=w201) -> ()  [unwired: 2 in, 2 out]
        n168 = local read "stop"() -> (w207:bool)
      }
    }
    frame Enabled {
    }
  }
  n169 = disable-structure shown="Enabled" {
    frame Disabled {
    }
    frame Enabled {
      n170 = local write "stop"(FALSE ("Boolean")) -> ()
    }
  }
  n171 = while {
    i -> [w231]
    stop <- w215 stop-if-true
    # "Основной цикл, измерения ПКТ-8 2"
    n172 = Equal?(x=w231, y=1) -> (x = y?=w232:bool)
    n173 = Or(x=w232, y="connect 2") -> (x .or. y?=w229:bool)
    n174 = case shown="True" w229 {
      tunnel: [_ w245] -> w227
      tunnel: [w243 w246] -> w230
      frame False {
        n175 = local read "connection ID 2"() -> (w243:refnum<k5>)
      }
      frame True {
        n176 = local write "disconnected 2"(FALSE ("disconnected")) -> ()
        n177 = TCP Open Connection(address="IP-адрес 2", remote port or service name="порт 2", timeout ms (60000)=2000) -> (connection ID=w246:refnum<k5>, error out=w245:errorcluster)  [unwired: 1 in, 1 out]
        "connection ID 2" <- w246
      }
    }
    n178 = Wait Until Next ms Multiple(millisecond multiple=u32 10) -> ()  [unwired: 1 out]
    n179 = local read "Configuring ADC?"() -> (w221:bool)
    n180 = case shown="False" w221 {
      tunnel: [w251 w417] -> w218
      tunnel: w227 -> [w311 w417]
      tunnel: w230 -> [w310 _]
      tunnel: [w252 w417] -> w219
      frame False {
        # "Есть синхронизация, \nвычитываем 10 байт данных"
        # "Проверка id канала"
        # "Синхронизация посылки \nизмерений канала АЦП\nформат посылки:\n000000000\\n"
        n181 = TCP Read(connection ID=w310, bytes to read=1, error in (no error)=w311, 7:T7."Immediate" ("mode (standard)"), 9:1000 ("timeout ms (25000)")) -> (connection ID out=w312:refnum<k5>, data out=w313:string, error out=w303:errorcluster)
        n182 = Match Pattern(string=w313, regular expression="\n") -> (offset past match=w309:i32)  [unwired: 4 out]
        n183 = case shown="1" w309 {
          tunnel: [w410 w416] -> w252
          tunnel: [_ w411] -> w304
          tunnel: w312 -> [_ w415]
          tunnel: w303 -> [w410 w414]
          frame -1, Default {
          }
          frame 1 {
            n184 = TCP Read(connection ID=w415, bytes to read=10, error in (no error)=w414, 9:5000 ("timeout ms (25000)")) -> (data out=w411:string, error out=w416:errorcluster)  [unwired: 2 out]
          }
        }
        n185 = call "String_match (SubVI).vi"("channel id"="^a" ("regular expression"), "input string"=w304, "error in"=w252) -> ("match ?"=w301:i32, "output string"=w298:string, "match substring"=w299:string, "error out"=w300:errorcluster)  [unwired: 13 in]
        n186 = case shown="1, Default" w301 {
          tunnel: [w403 w409] -> w282
          tunnel: w300 -> [w403 w408]
          tunnel: w299 -> [_ w406]
          tunnel: [w402 _] -> w316
          tunnel: w298 -> [w402 _]
          frame -1 {
          }
          frame 1, Default {
            n187 = call "Volts_to_temperature_(SubVI).vi"("ch_data_string"=w406, "error in"=w408) -> ("s? color"=w404:u32, "T solvation"=→"T9":dbl, "meas_voltage"=→"R9":dbl, "error out"=w409:errorcluster)  [unwired: 21 in, 1 out]
            n188 = property on="R9" class="DigNum (strict)"("NumText.TextColor"=w404) -> ()  [unwired: 2 in, 2 out]
          }
        }
        n189 = call "String_match (SubVI).vi"("channel id"="^b" ("regular expression"), "input string"=w316, "error in"=w282) -> ("match ?"=w296:i32, "output string"=w293:string, "match substring"=w294:string, "error out"=w295:errorcluster)  [unwired: 13 in]
        n190 = case shown="1, Default" w296 {
          tunnel: [w394 w401] -> w281
          tunnel: w295 -> [w394 w400]
          tunnel: w294 -> [_ w399]
          tunnel: w293 -> [w393 _]
          tunnel: [w393 _] -> w315
          frame -1 {
          }
          frame 1, Default {
            n191 = call "Volts_to_temperature_(SubVI).vi"("ch_data_string"=w399, "error in"=w400, "koeff. cluster"="T10 koeff.") -> ("s? color"=w396:u32, "T solvation"=→"T10":dbl, "meas_voltage"=→"R10":dbl, "error out"=w401:errorcluster)  [unwired: 20 in, 1 out]
            n192 = property on="R10" class="DigNum (strict)"("NumText.TextColor"=w396) -> ()  [unwired: 2 in, 2 out]
          }
        }
        n193 = call "String_match (SubVI).vi"("channel id"="^c" ("regular expression"), "input string"=w315, "error in"=w281) -> ("match ?"=w290:i32, "output string"=w289:string, "match substring"=w288:string, "error out"=w292:errorcluster)  [unwired: 13 in]
        n194 = case shown="1, Default" w290 {
          tunnel: w292 -> [w385 w392]
          tunnel: [w385 w391] -> w280
          tunnel: [w384 _] -> w314
          tunnel: w289 -> [w384 _]
          tunnel: w288 -> [_ w390]
          frame -1 {
          }
          frame 1, Default {
            n195 = call "Volts_to_temperature_(SubVI).vi"("ch_data_string"=w390, "error in"=w392, "koeff. cluster"="T11 koeff.") -> ("s? color"=w387:u32, "T solvation"=→"T11":dbl, "meas_voltage"=→"R11":dbl, "error out"=w391:errorcluster)  [unwired: 20 in, 1 out]
            n196 = property on="R11" class="DigNum (strict)"("NumText.TextColor"=w387) -> ()  [unwired: 2 in, 2 out]
          }
        }
        n197 = call "String_match (SubVI).vi"("channel id"="^d" ("regular expression"), "input string"=w314, "error in"=w280) -> ("match ?"=w285:i32, "output string"=w283:string, "match substring"=w284:string, "error out"=w286:errorcluster)  [unwired: 13 in]
        n198 = case shown="1, Default" w285 {
          tunnel: w286 -> [w376 w383]
          tunnel: [w376 w382] -> w279
          tunnel: w284 -> [_ w380]
          tunnel: w283 -> [w375 _]
          tunnel: [w375 _] -> w278
          frame -1 {
          }
          frame 1, Default {
            n199 = call "Volts_to_temperature_(SubVI).vi"("ch_data_string"=w380, "error in"=w383, "koeff. cluster"="T12 koeff.") -> ("s? color"=w378:u32, "T solvation"=→"T12":dbl, "meas_voltage"=→"R12":dbl, "error out"=w382:errorcluster)  [unwired: 20 in, 1 out]
            n200 = property on="R12" class="DigNum (strict)"("NumText.TextColor"=w378) -> ()  [unwired: 2 in, 2 out]
          }
        }
        n201 = call "String_match (SubVI).vi"("channel id"="^e" ("regular expression"), "input string"=w278, "error in"=w279) -> ("match ?"=w257:i32, "output string"=w260:string, "match substring"=w259:string, "error out"=w258:errorcluster)  [unwired: 13 in]
        n202 = case shown="1, Default" w257 {
          tunnel: [w367 w374] -> w275
          tunnel: w258 -> [w367 w373]
          tunnel: w259 -> [_ w372]
          tunnel: [w366 _] -> w253
          tunnel: w260 -> [w366 _]
          frame -1 {
          }
          frame 1, Default {
            n203 = call "Volts_to_temperature_(SubVI).vi"("ch_data_string"=w372, "error in"=w373, "koeff. cluster"="T13 koeff.") -> ("s? color"=w369:u32, "T solvation"=→"T13":dbl, "meas_voltage"=→"R13":dbl, "error out"=w374:errorcluster)  [unwired: 20 in, 1 out]
            n204 = property on="R13" class="DigNum (strict)"("NumText.TextColor"=w369) -> ()  [unwired: 2 in, 2 out]
          }
        }
        n205 = call "String_match (SubVI).vi"("channel id"="^f" ("regular expression"), "input string"=w253, "error in"=w275) -> ("match ?"=w262:i32, "output string"=w265:string, "match substring"=w264:string, "error out"=w263:errorcluster)  [unwired: 13 in]
        n206 = case shown="1, Default" w262 {
          tunnel: [w359 w365] -> w276
          tunnel: w263 -> [w359 w364]
          tunnel: w264 -> [_ w363]
          tunnel: w265 -> [w358 _]
          tunnel: [w358 _] -> w254
          frame -1 {
          }
          frame 1, Default {
            n207 = call "Volts_to_temperature_(SubVI).vi"("ch_data_string"=w363, "error in"=w364) -> ("s? color"=w360:u32, "T solvation"=→"T14":dbl, "meas_voltage"=→"R14":dbl, "error out"=w365:errorcluster)  [unwired: 21 in, 1 out]
            n208 = property on="R14" class="DigNum (strict)"("NumText.TextColor"=w360) -> ()  [unwired: 2 in, 2 out]
          }
        }
        n209 = call "String_match (SubVI).vi"("channel id"="^g" ("regular expression"), "input string"=w254, "error in"=w276) -> ("match ?"=w268:i32, "output string"=w269:string, "match substring"=w270:string, "error out"=w266:errorcluster)  [unwired: 13 in]
        n210 = case shown="1, Default" w268 {
          tunnel: w266 -> [w351 w357]
          tunnel: [w351 w356] -> w277
          tunnel: [w350 _] -> w255
          tunnel: w269 -> [w350 _]
          tunnel: w270 -> [_ w355]
          frame -1 {
          }
          frame 1, Default {
            n211 = call "Volts_to_temperature_(SubVI).vi"("ch_data_string"=w355, "error in"=w357) -> ("s? color"=w352:u32, "T solvation"=→"T15":dbl, "meas_voltage"=→"R15":dbl, "error out"=w356:errorcluster)  [unwired: 21 in, 1 out]
            n212 = property on="R15" class="DigNum (strict)"("NumText.TextColor"=w352) -> ()  [unwired: 2 in, 2 out]
          }
        }
        n213 = call "String_match (SubVI).vi"("channel id"="^h" ("regular expression"), "input string"=w255, "error in"=w277) -> ("match ?"=w250:i32, "output string"=w274:string, "match substring"=w273:string, "error out"=w272:errorcluster)  [unwired: 13 in]
        n214 = case shown="1, Default" w250 {
          tunnel: w272 -> [w317 w341]
          tunnel: w273 -> [_ w340]
          tunnel: w274 -> [_ _]
          tunnel: [w317 w338] -> w251
          frame -1 {
          }
          frame 1, Default {
            n215 = call "Volts_to_temperature_(SubVI).vi"("ch_data_string"=w340, "error in"=w341) -> ("s? color"=w336:u32, "T solvation"=→"T16":dbl, "meas_voltage"=→"R16":dbl, "error out"=w338:errorcluster)  [unwired: 21 in, 1 out]
            n216 = property on="R16" class="DigNum (strict)"("NumText.TextColor"=w336) -> ()  [unwired: 2 in, 2 out]
            n217 = local read "R10"() -> (w334:dbl)
            n218 = local read "R11"() -> (w333:dbl)
            n219 = local read "R12"() -> (w332:dbl)
            n220 = local read "R13"() -> (w331:dbl)
            n221 = local read "T13"() -> (w326:dbl)
            n222 = local read "R14"() -> (w320:dbl)
            n223 = local read "R15"() -> (w319:dbl)
            n224 = local read "R16"() -> (w318:dbl)
            n225 = local read "T10"() -> (w329:dbl)
            n226 = local read "T11"() -> (w328:dbl)
            n227 = local read "T12"() -> (w327:dbl)
            n228 = local read "T14"() -> (w325:dbl)
            n229 = local read "T15"() -> (w324:dbl)
            n230 = local read "T16"() -> (w323:dbl)
            n231 = local read "R9"() -> (w335:dbl)
            n232 = local read "T9"() -> (w330:dbl)
            n233 = Bundle("R9"=w335, "R10"=w334, "R11"=w333, "R12"=w332, "R13"=w331, "R14"=w320, "R15"=w319, "R16"=w318) -> (w322:T9)  [unwired: 1 in]
            n234 = Bundle("T9"=w330, "T10"=w329, "T11"=w328, "T12"=w327, "T13"=w326, "T14"=w325, "T15"=w324, "T16"=w323) -> (w321:T10)  [unwired: 1 in]
            n235 = flat-sequence {
              tunnel: w322 -> [w343]
              tunnel: w321 -> [w342]
              frame #0 {
                "ПКТ2-R" <- w343
                "ПКТ2-T" <- w342
              }
              frame #1 {
                "PKT1 updated" <- TRUE ("PKT1 updated")
              }
            }
            n236 = disable-structure shown="Disabled" {
              frame Disabled {
                n237 = call "GraphForm (SubVI).vi"(8:FALSE ("Update gr"), 10:"Азотные температуры" ("Title")) -> (0:w345, 2:w348, 5:w347)  [unwired: 15 in]
              }
              frame Enabled {
              }
            }
          }
        }
      }
      frame True {
      }
    }
    n238 = local read "disconnected 2"() -> (w220:bool)
    n239 = case shown="False" w220 {
      tunnel: [w235 FALSE] -> w226
      tunnel: w219 -> [w234 _]
      frame False {
        n240 = Unbundle By Name(w234) -> ("status"=w236:bool)
        n241 = Not(x=w236) -> (.not. x?=w235:bool)
      }
      frame True {
      }
    }
    "Связь с прибором 2" <- w226
    n242 = local read "Связь с прибором 2"() -> (w223:bool)
    n243 = And(x="disconnect 2", y=w223) -> (x .and. y?=w224:bool)
    n244 = case shown="True" w224 {
      tunnel: w218 -> [w238 w242]
      tunnel: [w238 w241] -> w222
      frame False {
      }
      frame True {
        n245 = local read "connection ID 2"() -> (w239:refnum<k5>)
        n246 = TCP Close Connection(connection ID=w239, error in (no error)=w242) -> (error out=w241:errorcluster)  [unwired: 2 out]
        "disconnected 2" <- TRUE ("disconnected")
      }
    }
    n247 = local read "stop"() -> (w215:bool)
    n248 = call <vilib>:"General Error Handler.vi"("type of dialog (OK msg:1)"=u32 0 ("milliseconds to wait"), "error in (no error)"=w222) -> ()  [unwired: 14 out]
  }
  n249 = while {
    stop <- w427 stop-if-true
    w432 = T6 0 items=["no dialog", "OK message", "continue or stop message", "OK message + warnings", "continue/stop + warnings"] ("type of dialog (OK msg:1)")
    # "Сохр. в файл"
    n250 = local read "PKT2 updated"() -> (w429:bool)
    n251 = local read "PKT1 updated"() -> (w428:bool)
    n252 = Multiply(x=u32 60, y="Интервал сохр. в файл, мин") -> (x*y=w421:u32)
    n253 = To Double Precision Float(number=w421) -> (double precision float=w420:dbl)
    n254 = Wait Until Next ms Multiple(millisecond multiple=u32 10) -> ()  [unwired: 1 out]
    n255 = call "Elapsed Time"("Time Target (s)"=w420, "Auto Reset"=TRUE ("Reset"), "Set Start Time (s)"=0.0) -> ("Time has Elapsed"=w419:bool, "error out"=w418:errorcluster)  [unwired: 9 in, 6 out]
    n256 = And(x=w429, y=w428) -> (x .and. y?=w430:bool)
    n257 = case shown="True" w430 {
      tunnel: [_ w441] -> w431
      tunnel: w419 -> [_ w440]
      tunnel: w418 -> [_ w437]
      frame False {
      }
      frame True {
        n258 = local read "Sensor 2"() -> (w433:dbl)
        n259 = local read "Sensor 1"() -> (w434:dbl)
        n260 = local read "ПКТ1-T"() -> (w449:T2)
        n261 = local read "ПКТ2-T"() -> (w448:T2)
        n262 = local read "ПКТ1-R"() -> (w447:T2)
        n263 = local read "ПКТ2-R"() -> (w446:T2)
        n264 = case shown="False" w440 {
          tunnel: w449 -> [w490 w504]
          tunnel: w448 -> [w489 w503]
          tunnel: w447 -> [w488 w502]
          tunnel: w446 -> [w487 w501]
          tunnel: [w490 w500] -> w445
          tunnel: [w489 w499] -> w444
          tunnel: [w488 w498] -> w443
          tunnel: [w487 w497] -> w442
          tunnel: [w486 w496] -> w441
          tunnel: w437 -> [w486 w495]
          tunnel: [w485 w494] -> w436
          tunnel: [w484 w493] -> w435
          tunnel: w434 -> [w485 w492]
          tunnel: w433 -> [w484 w491]
          frame False {
          }
          frame True {
            n265 = local read "File header exist?"() -> (w505:bool)
            n266 = case shown="False" w505 {
              tunnel: w504 -> [w513 w526]
              tunnel: w503 -> [w512 w525]
              tunnel: w502 -> [w511 w524]
              tunnel: w501 -> [w510 w523]
              tunnel: [w513 w526] -> w500
              tunnel: [w512 w525] -> w499
              tunnel: [w511 w524] -> w498
              tunnel: [w510 w523] -> w497
              tunnel: [w509 w521] -> w496
              tunnel: w495 -> [w508 w520]
              tunnel: [w507 w519] -> w494
              tunnel: [w506 w518] -> w493
              tunnel: w492 -> [w507 w519]
              tunnel: w491 -> [w506 w518]
              frame False {
                # "выполняется 1 раз"
                n267 = call "Ch_data_title_pattern 16 (SubVI).vi"("error in"=w508, "Единица измерений"="") -> ("error out"=w509:errorcluster, "Path"=→"Расположение файла":path, "Byte Stream File out"=→"refnum out":refnum<file>)  [unwired: 7 in]
                n268 = local write "File header exist?"(TRUE ("flag1")) -> ()
              }
              frame True {
                n269 = local read "refnum out"() -> (w522:refnum<file>)
                n270 = call "Ch_data_pattern_16_save (SubVI).vi"("error in"=w520, "R1-8 Cluster"=w524, "P S1"=w519, "T1-8 Cluster"=w526, "P S2"=w518, "R9-16"=w523, "T9-16"=w525, "file"=w522) -> ("error out"=w521:errorcluster)  [unwired: 19 in]
              }
            }
          }
        }
        n271 = local write "PKT2 updated"(FALSE ("PKT1 updated")) -> ()
        n272 = local write "PKT1 updated"(FALSE ("PKT1 updated")) -> ()
        n273 = Unbundle(w445) -> ("R1"=w450:dbl, "R2"=w451:dbl, "R3"=w452:dbl, "R4"=w453:dbl, "R5"=w454:dbl, "R6"=w455:dbl, "R7"=w456:dbl, "R8"=w457:dbl)
        n274 = Unbundle(w444) -> ("R1"=w458:dbl, "R2"=w459:dbl, "R3"=w460:dbl, "R4"=w461:dbl, "R5"=w462:dbl, "R6"=w463:dbl, "R7"=w464:dbl, "R8"=w465:dbl)
        n275 = Unbundle(w443) -> ("R1"=w482:dbl, "R2"=w481:dbl, "R3"=w480:dbl, "R4"=w479:dbl, "R5"=w478:dbl, "R6"=w477:dbl, "R7"=w476:dbl, "R8"=w475:dbl)
        n276 = Unbundle(w442) -> ("R1"=w474:dbl, "R2"=w473:dbl, "R3"=w472:dbl, "R4"=w471:dbl, "R5"=w470:dbl, "R6"=w469:dbl, "R7"=w468:dbl, "R8"=w467:dbl)
        n277 = Bundle("Sensor 1"=w436, "Sensor 2"=w435) -> ()  [unwired: 1 in, 1 out]
        n278 = Bundle("R1"=w450, "R2"=w451, "R3"=w452, "R4"=w453, "R5"=w454, "R6"=w455, "R7"=w456, "R8"=w457, "R1"=w458, "R2"=w459, "R3"=w460, "R4"=w461, "R5"=w462, "R6"=w463, "R7"=w464, "R8"=w465) -> (w466:T11)  [unwired: 1 in]
        n279 = Bundle("R1"=w482, "R2"=w481, "R3"=w480, "R4"=w479, "R5"=w478, "R6"=w477, "R7"=w476, "R8"=w475, "R1"=w474, "R2"=w473, "R3"=w472, "R4"=w471, "R5"=w470, "R6"=w469, "R7"=w468, "R8"=w467) -> (w483:T11)  [unwired: 1 in]
        n280 = global write "Global R.vi" "R"(w483) -> ()
        n281 = global write "Global T.vi" "T"(w466) -> ()
      }
    }
    n282 = local read "stop"() -> (w427:bool)
    n283 = call <vilib>:"General Error Handler.vi"("type of dialog (OK msg:1)"=w432, "error in (no error)"=w431) -> ()  [unwired: 9 in, 5 out]
  }
  n284 = while {
    i -> [w542]
    stop <- "stop" stop-if-true
    # "Основной цикл, измерения ПКТ-8 1"
    n285 = Equal?(x=w542, y=1) -> (x = y?=w543:bool)
    n286 = Or(x=w543, y="connect") -> (x .or. y?=w540:bool)
    n287 = case shown="True" w540 {
      tunnel: [_ w551] -> w538
      tunnel: [w550 w552] -> w541
      frame False {
        n288 = local read "connection ID"() -> (w550:refnum<k5>)
      }
      frame True {
        n289 = TCP Open Connection(address="IP-адрес", remote port or service name="порт", timeout ms (60000)=2000) -> (connection ID=w552:refnum<k5>, error out=w551:errorcluster)  [unwired: 1 in, 1 out]
        "connection ID" <- w552
      }
    }
    n290 = local read "Configuring ADC?"() -> (w532:bool)
    n291 = case shown="False" w532 {
      tunnel: [w557 w722] -> w530
      tunnel: w538 -> [w617 w722]
      tunnel: w541 -> [w616 _]
      tunnel: [w558 w722] -> w531
      frame False {
        # "Проверка id канала = a,\nсчитываем и проебразуем в Т\nсопротивление канала 1"
        # "Есть синхронизация, \nвычитываем 10 байт данных"
        # "Проверка id канала"
        # "Синхронизация посылки \nизмерений канала АЦП\nформат посылки:\n000000000\\n"
        n292 = TCP Read(connection ID=w616, bytes to read=1, error in (no error)=w617, 7:T7."Immediate" ("mode (standard)"), 9:1000 ("timeout ms (25000)")) -> (connection ID out=w618:refnum<k5>, data out=w619:string, error out=w609:errorcluster)
        n293 = Match Pattern(string=w619, regular expression="\n") -> (offset past match=w615:i32)  [unwired: 4 out]
        n294 = case shown="1" w615 {
          tunnel: [w715 w721] -> w558
          tunnel: [_ w716] -> w610
          tunnel: w618 -> [_ w720]
          tunnel: w609 -> [w715 w719]
          frame -1, Default {
          }
          frame 1 {
            n295 = TCP Read(connection ID=w720, bytes to read=10, error in (no error)=w719, 9:5000 ("timeout ms (25000)")) -> (data out=w716:string, error out=w721:errorcluster)  [unwired: 2 out]
          }
        }
        n296 = call "String_match (SubVI).vi"("channel id"="^a" ("regular expression"), "input string"=w610, "error in"=w558) -> ("match ?"=w607:i32, "output string"=w604:string, "match substring"=w605:string, "error out"=w606:errorcluster)  [unwired: 13 in]
        n297 = case shown="1, Default" w607 {
          tunnel: [w707 w714] -> w588
          tunnel: w606 -> [w707 w713]
          tunnel: w605 -> [_ w711]
          tunnel: [w706 _] -> w622
          tunnel: w604 -> [w706 _]
          frame -1 {
          }
          frame 1, Default {
            n298 = call "Volts_to_temperature_(SubVI).vi"("ch_data_string"=w711, "error in"=w713, "koeff. cluster"="T1 koeff.") -> ("s? color"=w709:u32, "T solvation"=→"Т1":dbl, "meas_voltage"=→"R1":dbl, "error out"=w714:errorcluster)  [unwired: 20 in, 1 out]
            n299 = property on="R1" class="DigNum (strict)"("NumText.TextColor"=w709) -> ()  [unwired: 2 in, 2 out]
          }
        }
        n300 = call "String_match (SubVI).vi"("channel id"="^b" ("regular expression"), "input string"=w622, "error in"=w588) -> ("match ?"=w602:i32, "output string"=w599:string, "match substring"=w600:string, "error out"=w601:errorcluster)  [unwired: 13 in]
        n301 = case shown="1, Default" w602 {
          tunnel: [w698 w705] -> w587
          tunnel: w601 -> [w698 w704]
          tunnel: w600 -> [_ w703]
          tunnel: w599 -> [w697 _]
          tunnel: [w697 _] -> w621
          frame -1 {
          }
          frame 1, Default {
            n302 = call "Volts_to_temperature_(SubVI).vi"("ch_data_string"=w703, "error in"=w704, "koeff. cluster"="T2 koeff.") -> ("s? color"=w700:u32, "T solvation"=→"Т2":dbl, "meas_voltage"=→"R2":dbl, "error out"=w705:errorcluster)  [unwired: 20 in, 1 out]
            n303 = property on="R2" class="DigNum (strict)"("NumText.TextColor"=w700) -> ()  [unwired: 2 in, 2 out]
          }
        }
        n304 = call "String_match (SubVI).vi"("channel id"="^c" ("regular expression"), "input string"=w621, "error in"=w587) -> ("match ?"=w596:i32, "output string"=w595:string, "match substring"=w594:string, "error out"=w598:errorcluster)  [unwired: 13 in]
        n305 = case shown="1, Default" w596 {
          tunnel: w598 -> [w689 w696]
          tunnel: [w689 w695] -> w586
          tunnel: [w688 _] -> w620
          tunnel: w595 -> [w688 _]
          tunnel: w594 -> [_ w694]
          frame -1 {
          }
          frame 1, Default {
            n306 = call "Volts_to_temperature_(SubVI).vi"("ch_data_string"=w694, "error in"=w696, "koeff. cluster"="T3 koeff.") -> ("s? color"=w691:u32, "T solvation"=→"Т3":dbl, "meas_voltage"=→"R3":dbl, "error out"=w695:errorcluster)  [unwired: 20 in, 1 out]
            n307 = property on="R3" class="DigNum (strict)"("NumText.TextColor"=w691) -> ()  [unwired: 2 in, 2 out]
          }
        }
        n308 = call "String_match (SubVI).vi"("channel id"="^d" ("regular expression"), "input string"=w620, "error in"=w586) -> ("match ?"=w591:i32, "output string"=w589:string, "match substring"=w590:string, "error out"=w592:errorcluster)  [unwired: 13 in]
        n309 = case shown="1, Default" w591 {
          tunnel: w592 -> [w680 w687]
          tunnel: [w680 w681] -> w585
          tunnel: w590 -> [_ w686]
          tunnel: w589 -> [w679 _]
          tunnel: [w679 _] -> w584
          frame -1 {
          }
          frame 1, Default {
            n310 = call "Volts_to_temperature_(SubVI) T4 !!!.vi"("ch_data_string"=w686, "error in"=w687, "koeff. cluster"="T4 koeff.") -> ("s? color"=w684:u32, "T solvation"=→"T4":dbl, "meas_voltage"=→"R4":dbl, "error out"=w681:errorcluster)  [unwired: 20 in, 1 out]
            n311 = property on="R4" class="DigNum (strict)"("NumText.TextColor"=w684) -> ()  [unwired: 2 in, 2 out]
          }
        }
        n312 = call "String_match (SubVI).vi"("channel id"="^e" ("regular expression"), "input string"=w584, "error in"=w585) -> ("match ?"=w563:i32, "output string"=w566:string, "match substring"=w565:string, "error out"=w564:errorcluster)  [unwired: 13 in]
        n313 = case shown="1, Default" w563 {
          tunnel: [w671 w678] -> w581
          tunnel: w564 -> [w671 w677]
          tunnel: w565 -> [_ w676]
          tunnel: [w670 _] -> w559
          tunnel: w566 -> [w670 _]
          frame -1 {
          }
          frame 1, Default {
            n314 = call "Volts_to_temperature_(SubVI).vi"("ch_data_string"=w676, "error in"=w677, "koeff. cluster"="T5 koeff.") -> ("s? color"=w673:u32, "T solvation"=→"Т5":dbl, "meas_voltage"=→"R5":dbl, "error out"=w678:errorcluster)  [unwired: 20 in, 1 out]
            n315 = property on="R5" class="DigNum (strict)"("NumText.TextColor"=w673) -> ()  [unwired: 2 in, 2 out]
          }
        }
        n316 = call "String_match (SubVI).vi"("channel id"="^f" ("regular expression"), "input string"=w559, "error in"=w581) -> ("match ?"=w568:i32, "output string"=w571:string, "match substring"=w570:string, "error out"=w569:errorcluster)  [unwired: 13 in]
        n317 = case shown="1, Default" w568 {
          tunnel: [w662 w669] -> w582
          tunnel: w569 -> [w662 w668]
          tunnel: w570 -> [_ w667]
          tunnel: w571 -> [w661 _]
          tunnel: [w661 _] -> w560
          frame -1 {
          }
          frame 1, Default {
            n318 = call "Volts_to_temperature_(SubVI).vi"("ch_data_string"=w667, "error in"=w668, "koeff. cluster"="T6 koeff.") -> ("s? color"=w664:u32, "T solvation"=→"Т6":dbl, "meas_voltage"=→"R6":dbl, "error out"=w669:errorcluster)  [unwired: 20 in, 1 out]
            n319 = property on="R6" class="DigNum (strict)"("NumText.TextColor"=w664) -> ()  [unwired: 2 in, 2 out]
          }
        }
        n320 = call "String_match (SubVI).vi"("channel id"="^g" ("regular expression"), "input string"=w560, "error in"=w582) -> ("match ?"=w574:i32, "output string"=w575:string, "match substring"=w576:string, "error out"=w572:errorcluster)  [unwired: 13 in]
        n321 = case shown="1, Default" w574 {
          tunnel: w572 -> [w653 w660]
          tunnel: [w653 w659] -> w583
          tunnel: [w652 _] -> w561
          tunnel: w575 -> [w652 _]
          tunnel: w576 -> [_ w658]
          frame -1 {
          }
          frame 1, Default {
            n322 = call "Volts_to_temperature_(SubVI).vi"("ch_data_string"=w658, "error in"=w660, "koeff. cluster"="T7 koeff.") -> ("s? color"=w655:u32, "T solvation"=→"Т7":dbl, "meas_voltage"=→"R7":dbl, "error out"=w659:errorcluster)  [unwired: 20 in, 1 out]
            n323 = property on="R7" class="DigNum (strict)"("NumText.TextColor"=w655) -> ()  [unwired: 2 in, 2 out]
          }
        }
        n324 = call "String_match (SubVI).vi"("channel id"="^h" ("regular expression"), "input string"=w561, "error in"=w583) -> ("match ?"=w556:i32, "output string"=w580:string, "match substring"=w579:string, "error out"=w578:errorcluster)  [unwired: 13 in]
        n325 = case shown="1, Default" w556 {
          tunnel: w578 -> [w623 w648]
          tunnel: w579 -> [_ w647]
          tunnel: w580 -> [_ _]
          tunnel: [w623 w642] -> w557
          frame -1 {
          }
          frame 1, Default {
            # "Все 8 каналов \nпрочитаны,\nвыводим показания \nна графики и \nсохраняем в файл"
            n326 = call "Volts_to_temperature_(SubVI).vi"("ch_data_string"=w647, "error in"=w648, "koeff. cluster"="T8 koeff.") -> ("s? color"=w644:u32, "T solvation"=→"Т8":dbl, "meas_voltage"=→"R8":dbl, "error out"=w642:errorcluster)  [unwired: 20 in, 1 out]
            n327 = property on="R8" class="DigNum (strict)"("NumText.TextColor"=w644) -> ()  [unwired: 2 in, 2 out]
            n328 = local read "R2"() -> (w640:dbl)
            n329 = local read "R3"() -> (w639:dbl)
            n330 = local read "R4"() -> (w638:dbl)
            n331 = local read "R7"() -> (w635:dbl)
            n332 = local read "R1"() -> (w641:dbl)
            n333 = local read "R5"() -> (w637:dbl)
            n334 = local read "Т1"() -> (w634:dbl)
            n335 = local read "Т5"() -> (w630:dbl)
            n336 = local read "R6"() -> (w626:dbl)
            n337 = local read "R8"() -> (w636:dbl)
            n338 = local read "Т2"() -> (w633:dbl)
            n339 = local read "Т3"() -> (w632:dbl)
            n340 = local read "T4"() -> (w631:dbl)
            n341 = local read "Т6"() -> (w629:dbl)
            n342 = local read "Т7"() -> (w628:dbl)
            n343 = local read "Т8"() -> (w627:dbl)
            n344 = Bundle("R1"=w641, "R2"=w640, "R3"=w639, "R4"=w638, "R5"=w637, "R6"=w626, "R7"=w635, "R8"=w636) -> (w625:T2)  [unwired: 1 in]
            n345 = Bundle("Т1"=w634, "Т2"=w633, "Т3"=w632, "T4"=w631, "Т5"=w630, "Т6"=w629, "Т7"=w628, "Т8"=w627) -> (w624:T12)  [unwired: 1 in]
            n346 = flat-sequence {
              tunnel: w625 -> [w650]
              tunnel: w624 -> [w649]
              frame #0 {
                "ПКТ1-R" <- w650
                "ПКТ1-T" <- w649
              }
              frame #1 {
                "PKT2 updated" <- TRUE ("PKT1 updated")
              }
            }
          }
        }
      }
      frame True {
      }
    }
    n347 = Unbundle By Name(w531) -> ("status"=w527:bool)
    n348 = Not(x=w527) -> (.not. x?=→"Связь с прибором":bool)
    n349 = Wait Until Next ms Multiple(millisecond multiple=u32 10) -> ()  [unwired: 1 out]
    n350 = local read "Связь с прибором"() -> (w534:bool)
    n351 = And(x="disconnect", y=w534) -> (x .and. y?=w535:bool)
    n352 = case shown="True" w535 {
      tunnel: w530 -> [w546 w549]
      tunnel: [w546 w548] -> w533
      frame False {
      }
      frame True {
        n353 = local read "connection ID"() -> (w547:refnum<k5>)
        n354 = TCP Close Connection(connection ID=w547, error in (no error)=w549) -> (error out=w548:errorcluster)  [unwired: 2 out]
      }
    }
    n355 = call <vilib>:"General Error Handler.vi"("type of dialog (OK msg:1)"=u32 0 ("milliseconds to wait"), "error in (no error)"=w533) -> ()  [unwired: 14 out]
  }
  n356 = disable-structure shown="Disabled" {
    frame Disabled {
      n357 = Open VI Reference() -> (vi path=w724:path, vi reference=w731:refnum<vi>, error out=w725:errorcluster)  [unwired: 5 in]
      n358 = invoke on="Invoke Node" class="VI" method="FP.Open"(reference=w731, error in=w725, "Activate"=TRUE ("Activate?"), "State"=T13."Standard") -> (reference out=w734:refnum<vi>, error out=w733:errorcluster)  [unwired: 1 in, 3 out]
      n359 = invoke on="Invoke Node" class="VI" method="Run VI"(reference=w734, error in=w733, "Wait until done"=TRUE ("Wait Until Done"), "Auto Dispose Ref"=FALSE ("Auto Dispose Reference")) -> (reference out=w726:refnum<vi>, error out=w732:errorcluster)  [unwired: 1 in, 3 out]
      n360 = Close Reference(reference=w726, error in (no error)=w732) -> (error out=w723:errorcluster)
      n361 = call <vilib>:"Simple Error Handler.vi"("error in (no error)"=w723) -> ()  [unwired: 4 in, 5 out]
    }
    frame Enabled {
    }
  }
